vi "Create Python Orchestration Script.vi"(7 "Override Address":bool, 8 "error in":errorcluster, 9 "Default Address":string, 10 "Configuration File Name":string="orchestration.py", 11 "Filtered Config Entries":string="1737340154015584000\ttest\tCreate\tTemplatePlugin.0.2.3.lvlibp:TemplatePlugin.lvclass\t<version> 0.2.3.0\t\n1737340198541890000\ttest\tConfigure\t{\"Common\":{\"Period (s)\":0.001,\"Offset (us)\":0,\"ClockID\":0,\"Priority\":101,\"Processor\":-2},\"Step\":100}\n1737340326509796000\tlovingit6\tCreate\tCIFCorePlugin.0.1.2.lvlibp:CIFCorePlugin.lvclass\t<version> 0.1.2.0\t\n1737340326559504000\tchannelme\tCreate\tTemplatePlugin.0.2.3.lvlibp:TemplatePlugin.lvclass\t<version> 0.2.3.0\t\n1737340326827852000\tchannelme\tConnect\t<publisher> channelme/doubleout <subscriber> channelme/doublein1 <data> \n1737340326835711000\tchannelme\tConfigure\t{\"Common\":{\"Period (s)\":0.001,\"Offset (us)\":0,\"ClockID\":0,\"Priority\":101,\"Processor\":-2},\"Step\":100}\n1737340327017380000\tlovingit6\tRun\n") -> (0 "error out":errorcluster, 2 "Orchestration File Path":path, 3 "Python Orchestration File":string)   [LabVIEW 2021, in "Python Orchestration.lvlib"]
uses:
  Python Orchestration.lvlib
  CIFConfigurationFile/CIF Configuration File.lvlib
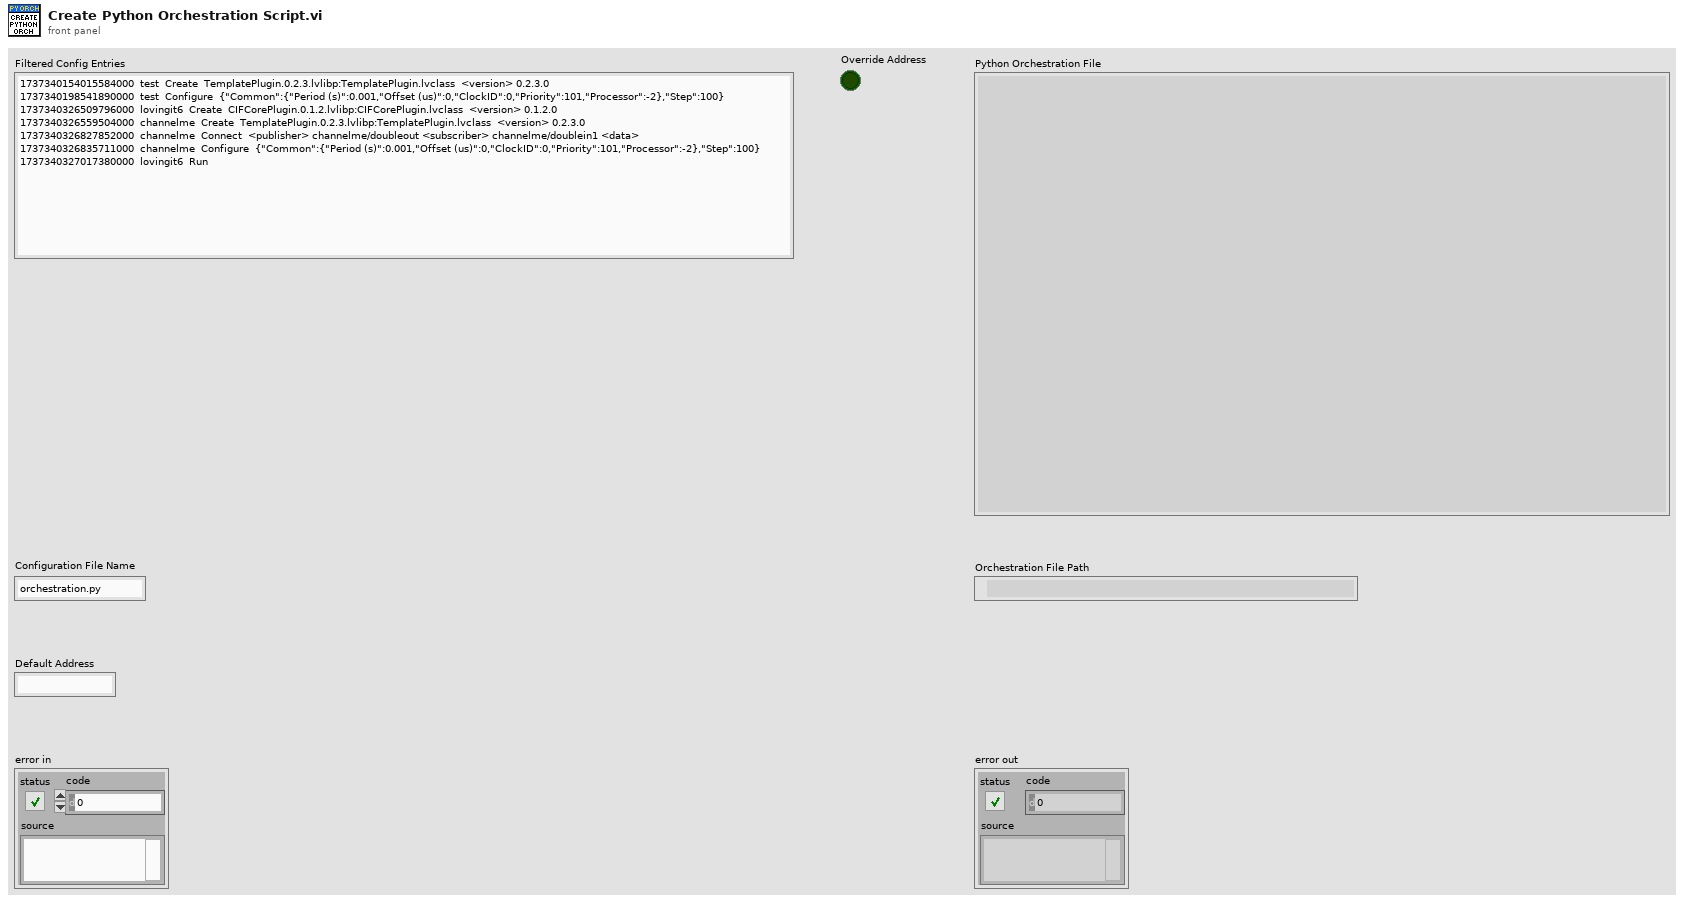
[diagram p1: front panel]
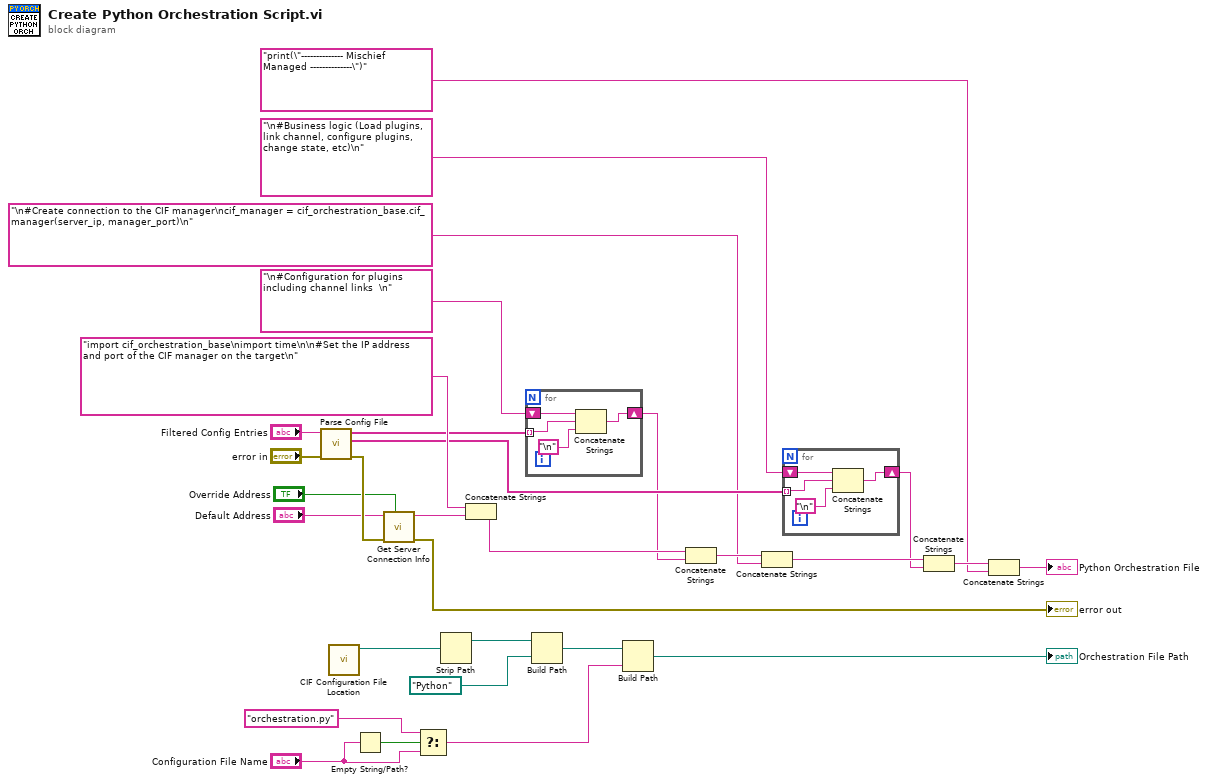
[diagram p0: block diagram]
diagram:
  n1 = call "Parse Config File.vi"("error in (no error)"="error in", "Filtered Config Entries"="Filtered Config Entries") -> ("error out"=w26:errorcluster, "Logic Entries"=w22:string[], "Configuration Entries"=w25:string[])  [unwired: 7 in]
  n2 = call "CIF Configuration File Location.vi"() -> ("configuration file path"=w11:path)  [unwired: 11 in]
  n3 = Empty String/Path?(string/path="Configuration File Name") -> (empty?=w4:bool)
  n4 = call "Get Server Connection Info.vi"("Override Address"="Override Address", "error in"=w26, "Default Address"="Default Address") -> ("error out"=→"error out":errorcluster, "Server Connection"=w28:string)  [unwired: 7 in]
  n5 = Select(t="orchestration.py" ("Configuration File Name 2"), s=w4, f="Configuration File Name") -> (s? t:f=w1:string)
  n6 = Strip Path(path=w11) -> (stripped path=w10:path)  [unwired: 1 out]
  n7 = Concatenate Strings("import cif_orchestration_base\nimport time\n\n#Set the IP address and port of the CIF manager on the target\n", w28) -> (w21:string)
  n8 = for {
    tunnel: w25 -> [w33] mode=indexing
    shift-right: [w32] -> w13
    shift-left: "\n#Configuration for plugins including channel links  \n" -> [w34]
    n9 = Concatenate Strings(w34, w33, "\n") -> (w32:string)
  }
  n10 = Build Path(base path=w10, name or relative path=path "Python" ("base path")) -> (appended path=w8:path)
  n11 = Build Path(base path=w8, name or relative path=w1) -> (appended path=→"Orchestration File Path":path)
  n12 = Concatenate Strings(w21, w13) -> (w20:string)
  n13 = Concatenate Strings(w20, "\n#Create connection to the CIF manager\ncif_manager = cif_orchestration_base.cif_manager(server_ip, manager_port)\n") -> (w18:string)
  n14 = for {
    tunnel: w22 -> [w37] mode=indexing
    shift-right: [w36] -> w17
    shift-left: "\n#Business logic (Load plugins, link channel, configure plugins, change state, etc)\n" -> [w38]
    n15 = Concatenate Strings(w38, w37, "\n") -> (w36:string)
  }
  n16 = Concatenate Strings(w18, w17) -> (w16:string)
  n17 = Concatenate Strings(w16, "print(\"-------------- Mischief Managed --------------\")") -> (→"Python Orchestration File":string)
